vi "BPM_main__.vi"() -> ()   [LabVIEW 2015]
doc: "Профилометр BPM v1.42"
uses:
  <vilib>/NI/Modbus Library/API/Master/Modbus Master.lvclass
  <vilib>/Utility/error.llb/DialogType.ctl
  Load and Save Controls_LV2009.llb/RWC_Actions.ctl
panel:
  in  "Tab Control":enum32{"ИЗМЕРЕНИЯ", "Н 1", "Н 2"}(tab)
  in  "Уст. 0":bool
  in  "Сброс":bool
  out "time":string
  out "trig led":bool
  out "Период":u8
  out "Измерения":dbl[](array[numeric])
  out "П2":dbl format="%#.2f"
  in  "Т интегрирования, мкс":u16=30 min=10 max=800 step=10
  in  "Шкала измерений":enum16{"3 пКл", "6 пКл", "12 пКл"}(ring)=enum."12 пКл"
  in  "stop":bool
  in  "Q мин.":dbl=-100.0 min=-200.0 max=4000.0 step=1.0
  in  "Q макс.":dbl=4100.0 min=0.0 max=4200.0 step=1.0
  in  "Автошкала":bool
  out "empty arr":dbl[](array[numeric])
  out "П2Xz":dbl[](array[numeric])
  out "Связь":refnum<class "Modbus Master.lvclass">
  in  "Пароль":string
  in  "ID блока 1":u8=80
  in  "Порт":u16
  in  "IP":string
  out "zero lvl":dbl[](array[numeric])
  out "update graphs":bool=TRUE
  out "t2":timestamp
  out "П2 upd":bool
  out "X axis":i32[](array[numeric])
  out "связь с блоком":bool
  out "Измерения в отсчетах АЦП":cluster{"X axis":i32[], "X1":dbl[]}[](graph) caption="gX1"
  # "Измерения"
  # "сек."
  # "Сумма"
  # "отсчеты"
  # "Конфигурация изм."
  # "Шкала"
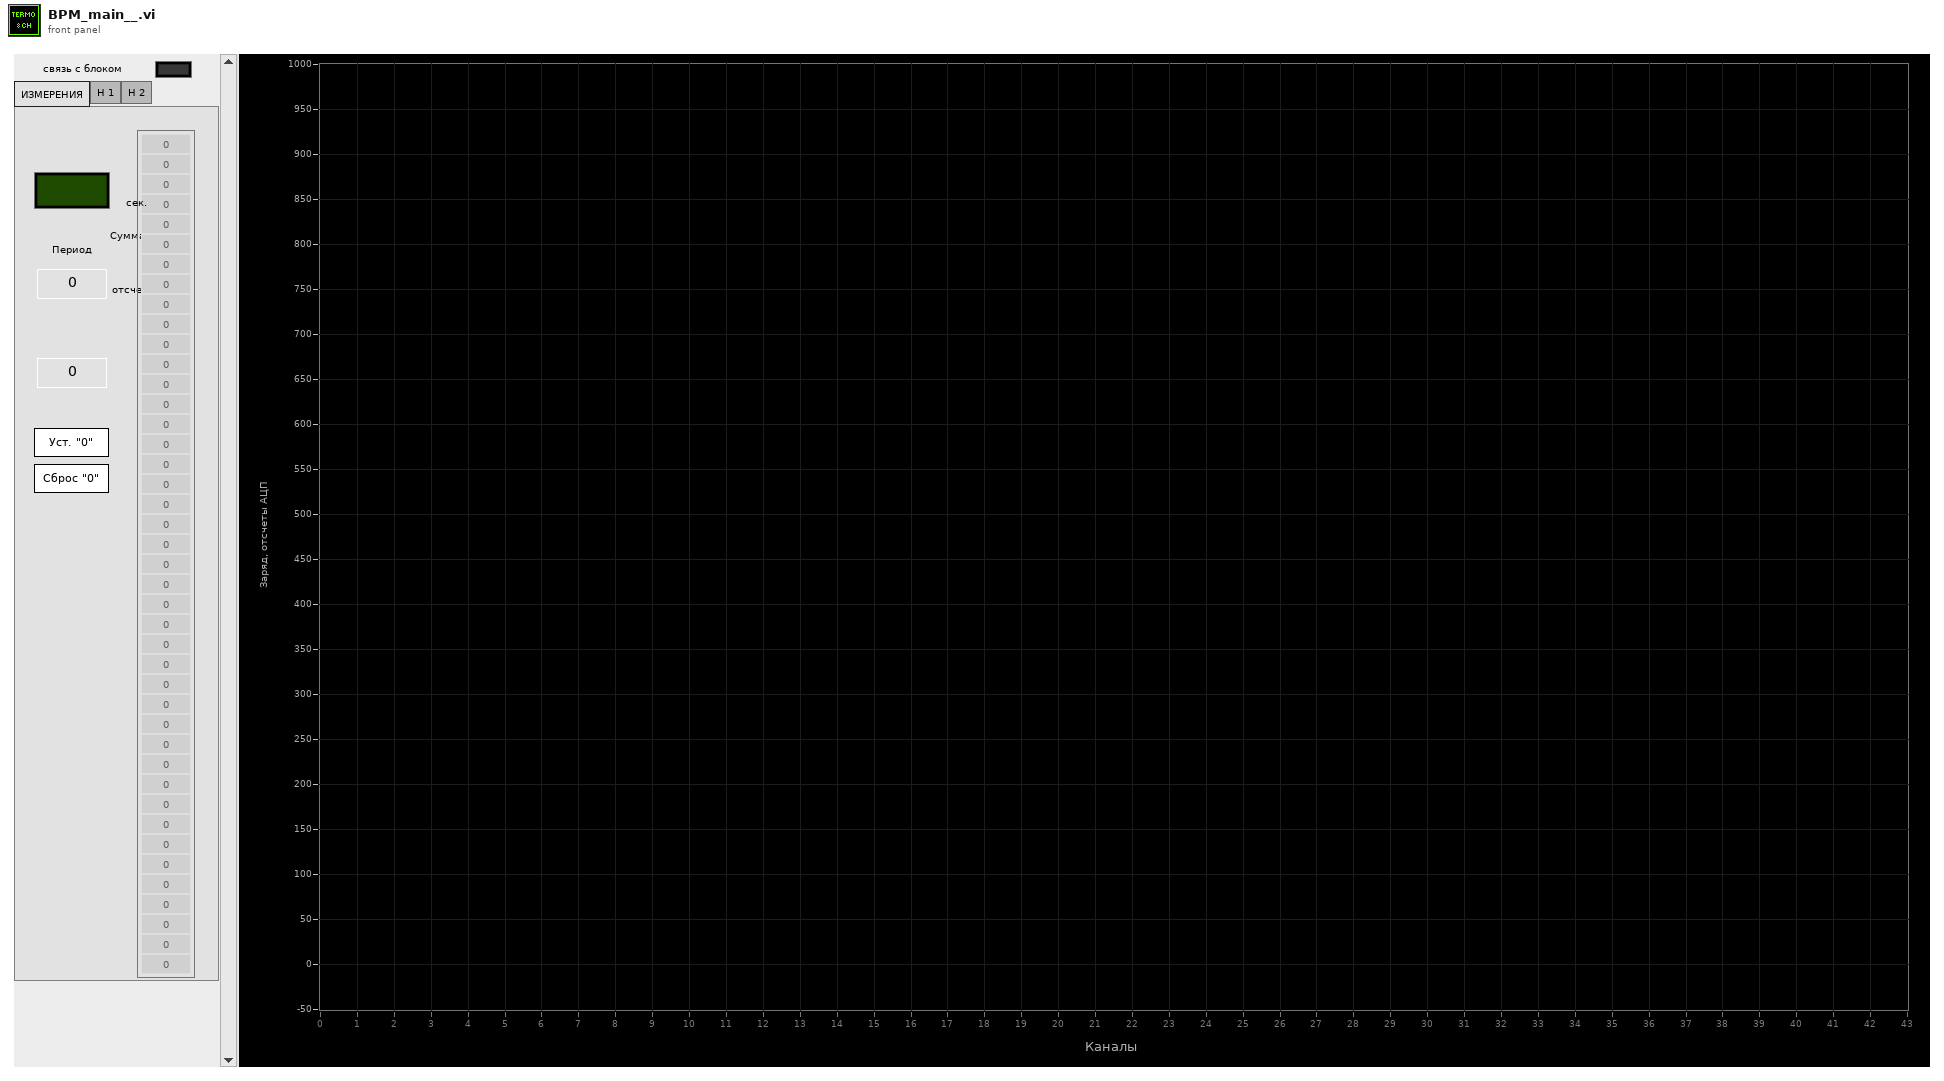
[diagram p1: front panel]
types:
  T1 = typedef "DialogType.ctl" = u16
  T2 = typedef "RWC_Actions.ctl" = enum16{"Read", "Write", "Read and Create"}
  T3 = enum8{"Enabled", "Disabled", "Disabled and Grayed Out"}
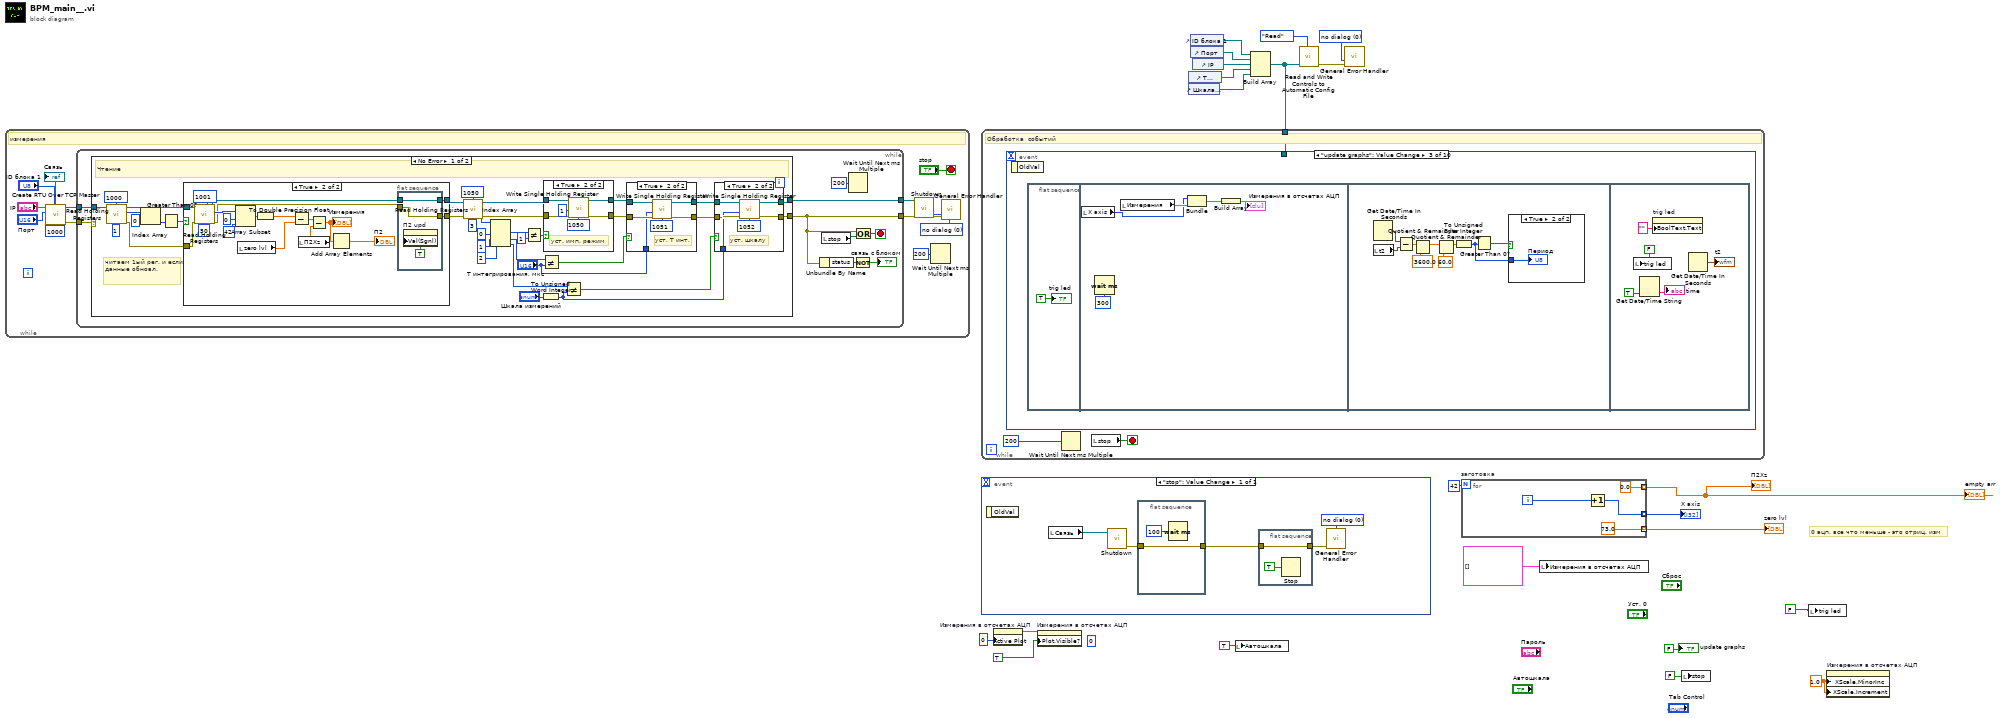
[diagram p0: block diagram]
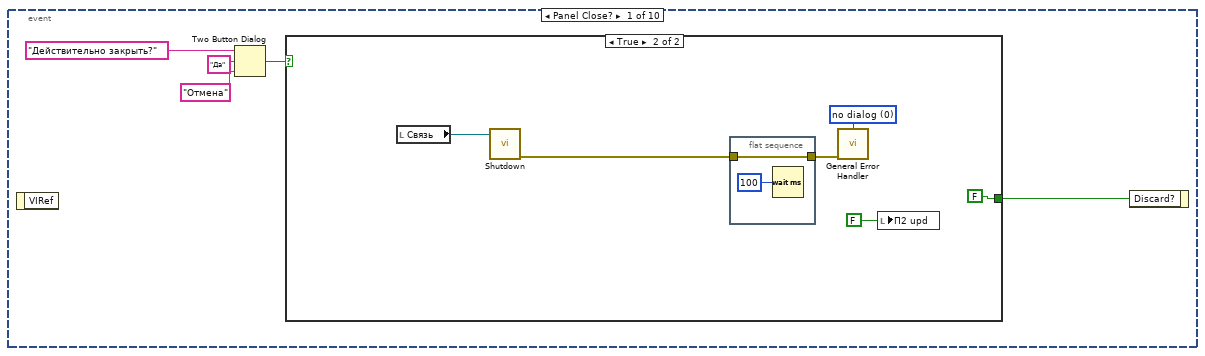
[diagram p2: hidden frame]
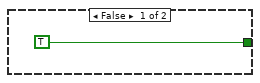
[diagram p3: hidden frame]
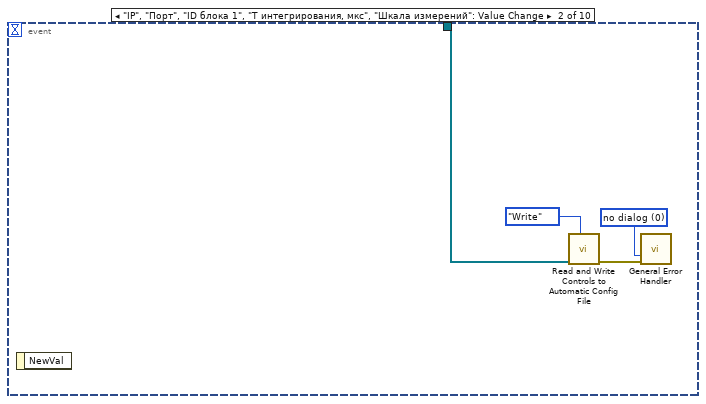
[diagram p4: hidden frame]
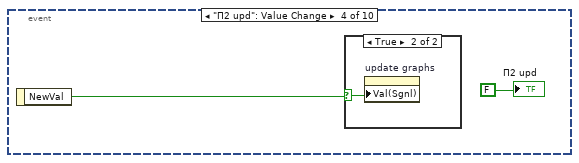
[diagram p6: hidden frame]
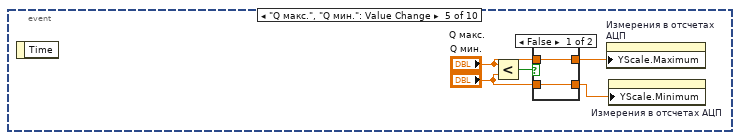
[diagram p8: hidden frame]
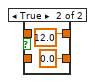
[diagram p9: hidden frame]
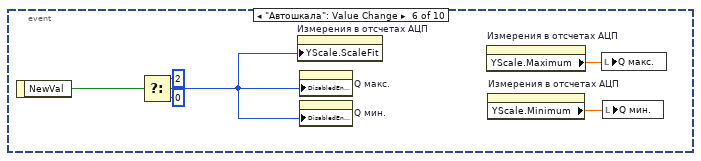
[diagram p10: hidden frame]
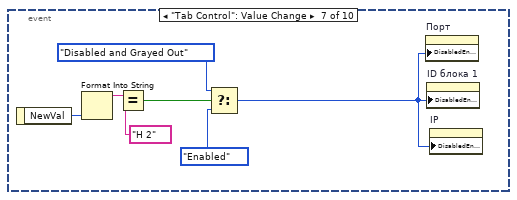
[diagram p11: hidden frame]
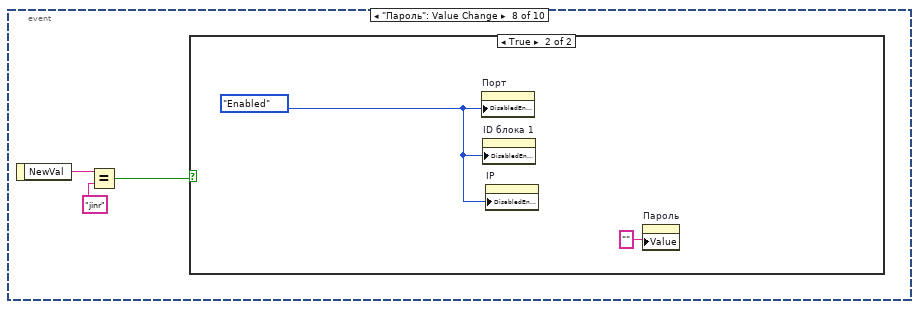
[diagram p12: hidden frame]
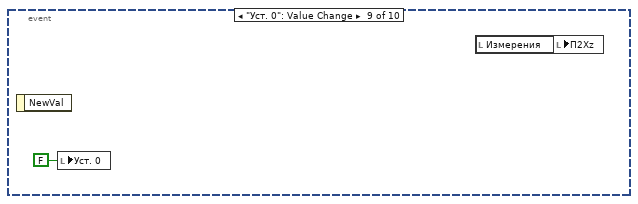
[diagram p14: hidden frame]
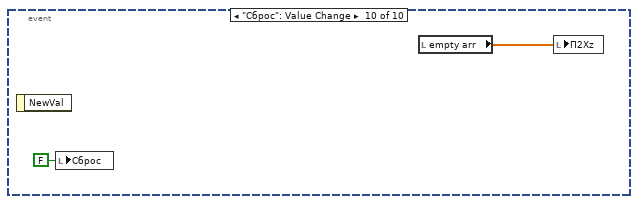
[diagram p15: hidden frame]
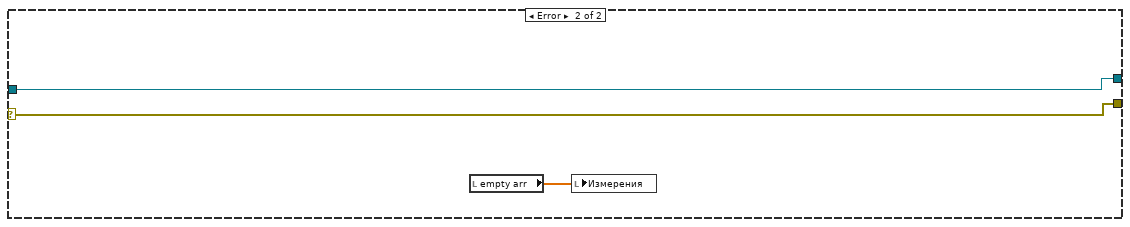
[diagram p20: hidden frame]
diagram:
  w9 = T1 0 items=["no dialog", "OK message", "continue or stop message", "OK message + warnings", "continue/stop + warnings"] ("type of dialog (OK msg:1)")
  (unwired) u32 0 ("Active Plot")
  w16 = 1.0 ("X Scale.Range:Increment")
  # "0 ацп, все что меньше - это отриц. изм"
  n1 = while {
    stop <- "stop" stop-if-true
    w24 = T1 0 items=["no dialog", "OK message", "continue or stop message", "OK message + warnings", "continue/stop + warnings"] ("type of dialog (OK msg:1)")
    # "измерения"
    n2 = call "Create RTU Over TCP Master.vi"("unit ID"="ID блока 1", "connect timeout ms"=1000, "port (502)"="Порт", "address"="IP") -> ("error out"=w28:errorcluster, "TCP master instance"=w29:refnum<class "Modbus Master.lvclass">)  [unwired: 6 in]
    "Связь" <- w29
    n3 = while {
      tunnel: w29 -> [w43]
      tunnel: w28 -> [w42]
      tunnel: [w36] -> w27
      tunnel: [w41] -> w26
      stop <- w39 stop-if-true
      n4 = case shown="No Error" w42 {
        selector: w42 -> [_ w127]
        tunnel: w43 -> [w76 w128]
        tunnel: [w54 w127] -> w36
        tunnel: [w55 w128] -> w41
        frame No Error {
          # "читаем 1ый рег. и если данные обновл."
          # "Чтение"
          n5 = call-dynamic "Read Holding Registers.vi"("number of inputs"=u16 1, "starting address"=u16 1000, "Modbus master in"=w76) -> ("error out"=w70:errorcluster, "register values"=w75:u16[], "Modbus master out"=w71:refnum<class "Modbus Master.lvclass">)  [unwired: 6 in]
          n6 = Index Array(array=w75, index=0) -> (element=w73:u16)
          n7 = Greater Than 0?(x=w73) -> (x > 0?=w72:bool)
          n8 = case shown="True" w72 {
            tunnel: w71 -> [w104 w120]
            tunnel: w70 -> [w103 w119]
            tunnel: [w104 w111] -> w67
            tunnel: [w103 w113] -> w66
            frame False {
            }
            frame True {
              n9 = call-dynamic "Read Holding Registers.vi"("error in"=w119, "number of inputs"=u16 50, "starting address"=u16 1001, "Modbus master in"=w120) -> ("error out"=w114:errorcluster, "register values"=w115:u16[], "Modbus master out"=w112:refnum<class "Modbus Master.lvclass">)  [unwired: 5 in]
              n10 = Array Subset(array=w115, index=0, length=42) -> (w116:u16[])
              n11 = local read "zero lvl"() -> (w108:dbl[])
              n12 = To Double Precision Float(number=w116) -> (double precision float=w110:dbl[])
              n13 = Subtract(x=w110, y=w108) -> (x-y=w109:dbl[])
              n14 = local read "П2Xz"() -> (w106:dbl[])
              n15 = Subtract(x=w109, y=w106) -> (x-y=w107:dbl[])
              "Измерения" <- w107
              n16 = Add Array Elements(numeric array=w107) -> (sum=→"П2":dbl)
              n17 = flat-sequence {
                tunnel: w114 -> [w125]
                tunnel: [w125] -> w113
                tunnel: w112 -> [w124]
                tunnel: [w124] -> w111
                frame #0 {
                  n18 = property on="П2 upd" class="Bool (strict)"("Val(Sgnl)"=TRUE ("dev 1 upd")) -> ()  [unwired: 2 in, 2 out]
                }
              }
            }
          }
          n19 = call-dynamic "Read Holding Registers.vi"("error in"=w66, "number of inputs"=u16 3, "starting address"=u16 1050, "Modbus master in"=w67) -> ("error out"=w62:errorcluster, "register values"=w64:u16[], "Modbus master out"=w65:refnum<class "Modbus Master.lvclass">)  [unwired: 5 in]
          n20 = Index Array(array=w64, index #1=0 ("index"), index #2=1 ("index"), index #3=2 ("index")) -> (element #1=w68:u16, element #2=w61:u16, element #3=w52:u16)
          n21 = Not Equal?(x=w68, y=u16 1) -> (x != y?=w69:bool)
          n22 = To Unsigned Word Integer(number="Шкала измерений") -> (unsigned 16bit integer=w49:u16)
          n23 = Not Equal?(x=w61, y="Т интегрирования, мкс") -> (x != y?=w53:bool)
          n24 = case shown="True" w69 {
            tunnel: [w96 w101] -> w60
            tunnel: [w95 w100] -> w59
            tunnel: w65 -> [w96 w99]
            tunnel: w62 -> [w95 w97]
            frame False {
            }
            frame True {
              # "уст. имп. режим"
              n25 = call-dynamic "Write Single Holding Register.vi"("error in"=w97, "register to write"=u16 1, "address"=u16 1050 ("starting address"), "Modbus master in"=w99) -> ("error out"=w100:errorcluster, "Modbus master out"=w101:refnum<class "Modbus Master.lvclass">)  [unwired: 6 in]
            }
          }
          n26 = Not Equal?(x=w52, y=w49) -> (x != y?=w51:bool)
          n27 = case shown="True" w53 {
            tunnel: [w88 w93] -> w58
            tunnel: [w87 w92] -> w57
            tunnel: w60 -> [w88 w91]
            tunnel: w59 -> [w87 w90]
            tunnel: "Т интегрирования, мкс" -> [_ w89]
            frame False {
            }
            frame True {
              # "уст. Т инт."
              n28 = call-dynamic "Write Single Holding Register.vi"("error in"=w90, "register to write"=w89, "address"=u16 1051 ("starting address"), "Modbus master in"=w91) -> ("error out"=w92:errorcluster, "Modbus master out"=w93:refnum<class "Modbus Master.lvclass">)  [unwired: 6 in]
            }
          }
          n29 = case shown="True" w51 {
            tunnel: [w80 w85] -> w55
            tunnel: [w79 w84] -> w54
            tunnel: w58 -> [w80 w83]
            tunnel: w57 -> [w79 w82]
            tunnel: w49 -> [_ w81]
            frame False {
            }
            frame True {
              # "уст. шкалу"
              n30 = call-dynamic "Write Single Holding Register.vi"("error in"=w82, "register to write"=w81, "address"=u16 1052 ("starting address"), "Modbus master in"=w83) -> ("error out"=w84:errorcluster, "Modbus master out"=w85:refnum<class "Modbus Master.lvclass">)  [unwired: 6 in]
            }
          }
        }
        frame Error {
          n31 = local read "empty arr"() -> (w126:dbl[])
          n32 = local write "Измерения"(w126) -> ()
        }
      }
      n33 = Unbundle By Name(w36) -> ("status"=w38:bool)
      n34 = local read "stop"() -> (w40:bool)
      n35 = Wait Until Next ms Multiple(millisecond multiple=u32 200) -> ()  [unwired: 1 out]
      n36 = Not(x=w38) -> (.not. x?=→"связь с блоком":bool)
      n37 = Or(x=w36, y=w40) -> (x .or. y?=w39:bool)
    }
    n38 = call-dynamic "Shutdown.vi"("error in"=w27, "Modbus master in"=w26) -> ("error out"=w25:errorcluster)  [unwired: 9 in]
    n39 = Wait Until Next ms Multiple(millisecond multiple=u32 200) -> ()  [unwired: 1 out]
    n40 = call <vilib>:"General Error Handler.vi"("type of dialog (OK msg:1)"=w24, "error in (no error)"=w25) -> ()  [unwired: 1 in, 13 out]
  }
  n41 = event shown="[0] \"stop\": Value Change" {
    selector: _ -> [_]
    dyn-events: _ -> [_]
    timeout: _ -> [_]
    event "stop": Value Change {
      w131 = T1 0 items=["no dialog", "OK message", "continue or stop message", "OK message + warnings", "continue/stop + warnings"] ("type of dialog (OK msg:1)")
      n42 = event-data() -> ()  [unwired: 1 in, 1 out]
      n43 = local read "Связь"() -> (w133:refnum<class "Modbus Master.lvclass">)
      n44 = call-dynamic "Shutdown.vi"("Modbus master in"=w133) -> ("error out"=w132:errorcluster)  [unwired: 10 in]
      n45 = flat-sequence {
        tunnel: w132 -> [w136]
        tunnel: [w136] -> w129
        frame #0 {
          n46 = Wait (ms)(milliseconds to wait=u32 100) -> ()  [unwired: 1 out]
        }
      }
      n47 = flat-sequence {
        tunnel: w129 -> [w135]
        tunnel: [w135] -> w130
        frame #0 {
          n48 = Stop(stop? (T)=TRUE) -> ()
        }
      }
      n49 = call <vilib>:"General Error Handler.vi"("error in (no error)"=w130, "[exception action] (none:0)"=w131) -> ()  [unwired: 2 in, 12 out]
    }
  }
  n50 = property on="Измерения в отсчетах АЦП" class="XYGraph (strict)"("Active Plot"=u32 0) -> (error out=w14:errorcluster)  [unwired: 2 in, 1 out]
  n51 = property on="Измерения в отсчетах АЦП" class="XYGraph (strict)"(error in=w14, "Plot.Visible?"=TRUE ("Plot.Visible")) -> ()  [unwired: 1 in, 2 out]
  n52 = control-ref of="Т интегрирования, мкс"() -> (w2:refnum<vi>)
  n53 = control-ref of="Шкала измерений"() -> (w1:refnum<vi>)
  n54 = control-ref of="ID блока 1"() -> (w7:refnum<vi>)
  n55 = control-ref of="Порт"() -> (w6:refnum<vi>)
  n56 = control-ref of="IP"() -> (w5:refnum<vi>)
  n57 = local write "Автошкала"(TRUE ("Автошкала")) -> ()
  n58 = Build Array(w7, w6, w5, w2, w1) -> (w4:refnum<vi>[])
  n59 = while {
    tunnel: w4 -> [w138]
    stop <- w139 stop-if-true
    # "Обработка  событий"
    n60 = event shown="[2] \"update graphs\": Value Change" {
      selector: _ -> [_ _ _ _ _ _ _ _ _ _]
      dyn-events: _ -> [_ _ _ _ _ _ _ _ _ _]
      timeout: _ -> [_ _ _ _ _ _ _ _ _ _]
      tunnel: w138 -> [_ w155 _ _ _ _ _ _ _ _]
      event Panel Close? {
        n61 = event-data() -> ()  [unwired: 2 out]
        n62 = Two Button Dialog(message="Действительно закрыть?", 1:"Отмена" ("T button name (\"OK\")"), 2:"Да" ("T button name (\"OK\")")) -> (T button?=w145:bool)
        n63 = case shown="True" w145 {
          tunnel: [TRUE ("Discard?") FALSE ("Discard?")] -> w141
          frame False {
          }
          frame True {
            w150 = T1 0 items=["no dialog", "OK message", "continue or stop message", "OK message + warnings", "continue/stop + warnings"] ("type of dialog (OK msg:1)")
            n64 = local read "Связь"() -> (w151:refnum<class "Modbus Master.lvclass">)
            n65 = call-dynamic "Shutdown.vi"("Modbus master in"=w151) -> ("error out"=w147:errorcluster)  [unwired: 10 in]
            n66 = flat-sequence {
              tunnel: w147 -> [w154]
              tunnel: [w154] -> w149
              frame #0 {
                n67 = Wait (ms)(milliseconds to wait=u32 100) -> ()  [unwired: 1 out]
              }
            }
            n68 = call <vilib>:"General Error Handler.vi"("error in (no error)"=w149, "[exception action] (none:0)"=w150) -> ()  [unwired: 2 in, 12 out]
            n69 = local write "П2 upd"(FALSE ("dev 1 upd")) -> ()
          }
        }
        n70 = event-data("Discard?"=w141) -> ()  [unwired: 1 in, 1 out]
      }
      event "IP", "Порт", "ID блока 1", "Т интегрирования, мкс", "Шкала измерений": Value Change {
        w157 = T1 0 items=["no dialog", "OK message", "continue or stop message", "OK message + warnings", "continue/stop + warnings"] ("type of dialog (OK msg:1)")
        n71 = event-data() -> ()  [unwired: 2 out]
        n72 = call "Read and Write Controls to Automatic Config File.vi"("Action"=RWC_Actions."Write", "Control References"=w155) -> ("error out"=w158:errorcluster)  [unwired: 9 in]
        n73 = call <vilib>:"General Error Handler.vi"("type of dialog (OK msg:1)"=w157, "error in (no error)"=w158) -> ()  [unwired: 1 in, 13 out]
      }
      event "update graphs": Value Change {
        n74 = event-data() -> ()  [unwired: 2 out]
        n75 = flat-sequence {
          frame #0 {
            "trig led" <- TRUE ("trig led")
          }
          frame #1 {
            n76 = local read "X axis"() -> (w161:i32[])
            n77 = Wait (ms)(milliseconds to wait=u32 300) -> ()  [unwired: 1 out]
            n78 = local read "Измерения"() -> (w163:dbl[])
            n79 = Bundle("X axis"=w161, "Измерения"=w163) -> (w164:cluster{"X axis":i32[], "Измерения":dbl[]})  [unwired: 1 in]
            n80 = Build Array(w164) -> (→"Измерения в отсчетах АЦП":cluster{"X axis":i32[], "Измерения":dbl[]}[])
          }
          frame #2 {
            n81 = Get Date/Time In Seconds() -> (seconds since 1Jan1904=w173:timestamp)
            n82 = local read "t2"() -> (w172:timestamp)
            n83 = Subtract(x=w173, y=w172) -> (x-y=w168:dbl)
            n84 = Quotient & Remainder(x=w168, y=3600.0 ("# sec/hour")) -> (x-y*floor(x/y)=w171:dbl)  [unwired: 1 out]
            n85 = Quotient & Remainder(x=w171, y=60.0 ("# sec/min")) -> (x-y*floor(x/y)=w167:dbl)  [unwired: 1 out]
            n86 = To Unsigned Byte Integer(number=w167) -> (unsigned 8bit integer=w165:u8)
            n87 = Greater Than 0?(x=w165) -> (x > 0?=w166:bool)
            n88 = case shown="True" w166 {
              tunnel: w165 -> [_ w174]
              frame False {
              }
              frame True {
                "Период" <- w174
              }
            }
          }
          frame #3 {
            n89 = local write "trig led"(FALSE ("обновл")) -> ()
            n90 = Get Date/Time String(want seconds? (F)=TRUE) -> (time string=→"time":string)  [unwired: 2 in, 1 out]
            n91 = property on="trig led" class="Bool (strict)"("BoolText.Text"="" ("Boolean Text.Text")) -> ()  [unwired: 2 in, 2 out]
            n92 = Get Date/Time In Seconds() -> (seconds since 1Jan1904=→"t2":timestamp)
          }
        }
      }
      event "П2 upd": Value Change {
        n93 = event-data() -> ("NewVal"=w180:bool)  [unwired: 1 out]
        n94 = case shown="True" w180 {
          selector: w180 -> [_ w182]
          frame False {
          }
          frame True {
            n95 = property on="update graphs" class="Bool (strict)"("Val(Sgnl)"=w182) -> ()  [unwired: 2 in, 2 out]
          }
        }
        "П2 upd" <- FALSE ("1П2 upd")
      }
      event "Q макс.", "Q мин.": Value Change {
        n96 = event-data() -> ()  [unwired: 2 out]
        n97 = Less?(x="Q макс.", y="Q мин.") -> (x < y?=w187:bool)
        n98 = case shown="False" w187 {
          tunnel: [w188 12.0 ("x+1")] -> w184
          tunnel: [w189 0.0 ("x+1")] -> w183
          tunnel: "Q макс." -> [w188 _]
          tunnel: "Q мин." -> [w189 _]
          frame False {
          }
          frame True {
          }
        }
        n99 = property on="Измерения в отсчетах АЦП" class="XYGraph (strict)"("YScale.Maximum"=w184) -> ()  [unwired: 2 in, 2 out]
        n100 = property on="Измерения в отсчетах АЦП" class="XYGraph (strict)"("YScale.Minimum"=w183) -> ()  [unwired: 2 in, 2 out]
      }
      event "Автошкала": Value Change {
        n101 = event-data() -> ("NewVal"=w195:bool)  [unwired: 1 out]
        n102 = Select(t=u8 2 ("Y Scale.Scale Fit"), s=w195, f=u8 0 ("Y Scale.Scale Fit")) -> (s? t:f=w192:u8)
        n103 = property on="Измерения в отсчетах АЦП" class="XYGraph (strict)"("YScale.ScaleFit"=w192) -> ()  [unwired: 2 in, 2 out]
        n104 = property on="Q макс." class="DigNum (strict)"("DisabledEnum"=w192) -> ()  [unwired: 2 in, 2 out]
        n105 = property on="Q мин." class="DigNum (strict)"("DisabledEnum"=w192) -> ()  [unwired: 2 in, 2 out]
        n106 = property on="Измерения в отсчетах АЦП" class="XYGraph (strict)"() -> ("YScale.Maximum"=w194:dbl)  [unwired: 2 in, 2 out]
        n107 = property on="Измерения в отсчетах АЦП" class="XYGraph (strict)"() -> ("YScale.Minimum"=w193:dbl)  [unwired: 2 in, 2 out]
        n108 = local write "Q макс."(w194) -> ()
        n109 = local write "Q мин."(w193) -> ()
      }
      event "Tab Control": Value Change {
        n110 = event-data() -> ("NewVal"=w204:enum32{"ИЗМЕРЕНИЯ", "Н 1", "Н 2"})  [unwired: 1 out]
        n111 = Format Into String(w204) -> (resulting string=w203:string)  [unwired: 3 in, 1 out]
        n112 = Equal?(x=w203, y="Н 2") -> (x = y?=w201:bool)
        n113 = Select(t=T3."Disabled and Grayed Out" ("Disabled"), s=w201, f=T3."Enabled" ("Disabled")) -> (s? t:f=w198:T3)
        n114 = property on="Порт" class="DigNum (strict)"("DisabledEnum"=w198) -> ()  [unwired: 2 in, 2 out]
        n115 = property on="ID блока 1" class="DigNum (strict)"("DisabledEnum"=w198) -> ()  [unwired: 2 in, 2 out]
        n116 = property on="IP" class="Str"("DisabledEnum"=w198) -> ()  [unwired: 2 in, 2 out]
      }
      event "Пароль": Value Change {
        n117 = event-data() -> ("NewVal"=w206:string)  [unwired: 1 out]
        n118 = Equal?(x=w206, y="jinr") -> (x = y?=w205:bool)
        n119 = case shown="True" w205 {
          frame False {
          }
          frame True {
            w208 = T3."Enabled" ("Disabled")
            n120 = property on="Порт" class="DigNum (strict)"("DisabledEnum"=w208) -> ()  [unwired: 2 in, 2 out]
            n121 = property on="ID блока 1" class="DigNum (strict)"("DisabledEnum"=w208) -> ()  [unwired: 2 in, 2 out]
            n122 = property on="IP" class="Str"("DisabledEnum"=w208) -> ()  [unwired: 2 in, 2 out]
            n123 = property on="Пароль" class="Str"("Value"="" ("Пароль")) -> ()  [unwired: 2 in, 2 out]
          }
        }
      }
      event "Уст. 0": Value Change {
        n124 = event-data() -> ()  [unwired: 2 out]
        n125 = local write "Уст. 0"(FALSE ("Уст. 0")) -> ()
        n126 = local read "Измерения"() -> (w210:dbl[])
        n127 = local write "П2Xz"(w210) -> ()
      }
      event "Сброс": Value Change {
        n128 = event-data() -> ()  [unwired: 2 out]
        n129 = local write "Сброс"(FALSE ("Уст. 0")) -> ()
        n130 = local read "empty arr"() -> (w212:dbl[])
        n131 = local write "П2Xz"(w212) -> ()
      }
    }
    n132 = Wait Until Next ms Multiple(millisecond multiple=u32 200) -> ()  [unwired: 1 out]
    n133 = local read "stop"() -> (w139:bool)
  }
  n134 = call "Read and Write Controls to Automatic Config File.vi"("Action"=RWC_Actions."Read", "Control References"=w4) -> ("error out"=w8:errorcluster)  [unwired: 9 in]
  n135 = call <vilib>:"General Error Handler.vi"("type of dialog (OK msg:1)"=w9, "error in (no error)"=w8) -> ()  [unwired: 1 in, 13 out]
  n136 = for "заготовка" {
    N: 42 -> [_]
    tunnel: [w214] -> w20 mode=indexing
    tunnel: [0.0] -> w12 mode=indexing
    tunnel: [73.0] -> w18 mode=indexing
    i -> [w215]
    n137 = Increment(x=w215) -> (x+1=w214:i32)
  }
  "X axis" <- w20
  "П2Xz" <- w12
  "empty arr" <- w12
  "zero lvl" <- w18
  n138 = local write "Измерения в отсчетах АЦП"(cluster{"X axis":i32[], "Измерения":dbl[]}[] [] ("appended array")) -> ()
  n139 = local write "stop"(FALSE ("Boolean")) -> ()
  n140 = local write "trig led"(FALSE ("обновл")) -> ()
  n141 = property on="Измерения в отсчетах АЦП" class="XYGraph (strict)"("XScale.MinorInc"=w16, "XScale.Increment"=w16) -> ()  [unwired: 2 in, 2 out]
  "update graphs" <- FALSE ("обновл")
